vi "ALTS-2015 Load VI Dynamically v1.0.vi"(5 "Auto Dispose Reference":bool=TRUE, 6 "Show FP?":bool=TRUE, 7 "Wait until done":bool, 8 "error in":errorcluster, 10 "VI Path":path) -> (0 "error out":errorcluster)   [LabVIEW 2013]
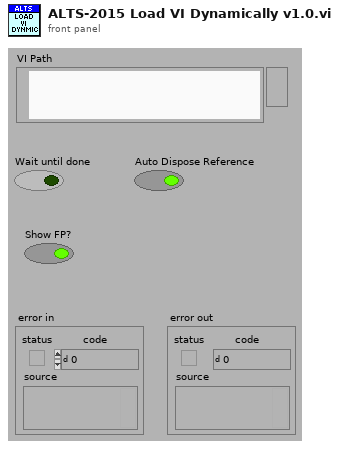
[diagram p1: front panel]
types:
  T1 = enum32{"Bad", "Idle", "Run top level", "Running"}
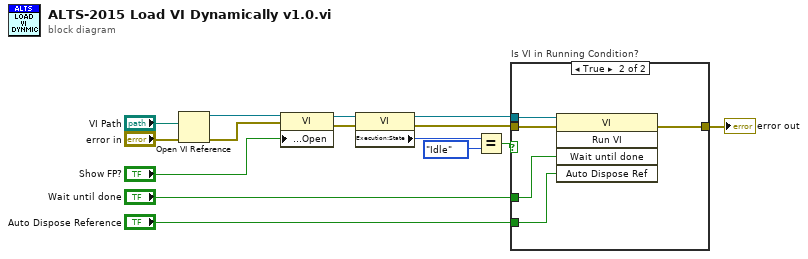
[diagram p0: block diagram]
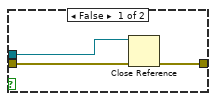
[diagram p2: hidden frame]
diagram:
  n1 = Open VI Reference(vi path="VI Path", error in (no error)="error in") -> (vi reference=w15:refnum<vi>, error out=w14:errorcluster)  [unwired: 4 in]
  n2 = property class="VI"(reference=w15, error in=w14, "Front Panel Window:Open"="Show FP?") -> (reference out=w13:refnum<vi>, error out=w12:errorcluster)
  n3 = property class="VI"(reference=w13, error in=w12) -> (reference out=w11:refnum<vi>, error out=w10:errorcluster, "Execution:State"=w9:T1)
  n4 = Equal?(x=w9, y=T1."Idle") -> (x = y?=w7:bool)
  n5 = case "Is VI in Running Condition?" shown="True" w7 {
    tunnel: w11 -> [w18 w23]
    tunnel: w10 -> [w17 w22]
    tunnel: [w16 w21] -> w1
    tunnel: "Wait until done" -> [_ w20]
    tunnel: "Auto Dispose Reference" -> [_ w19]
    frame False {
      n6 = Close Reference(reference=w18, error in (no error)=w17) -> (error out=w16:errorcluster)
    }
    frame True {
      n7 = invoke class="VI" method="Run VI"(reference=w23, error in=w22, "Wait until done"=w20, "Auto Dispose Ref"=w19) -> (error out=w21:errorcluster)  [unwired: 1 in, 4 out]
    }
  }
  "error out" <- w1
